vi "coler1.vi"(8 "error in":errorcluster, 11 "代刚":bool) -> (0 "error out":errorcluster)   [LabVIEW 2018]
uses:
  <vilib>/vision/NI_Vision_Development_Module.lvlib
panel:
  out "Array 3":dbl[](array[numeric])
  out "Color":u32(colorbox)
  out "Array":dbl[](array[numeric])
  out "Array 2":enum16{"黑", "紅", "黃", "綠", "藍"}[](array[ring])
  out "Image Out":T1(plugin-control)
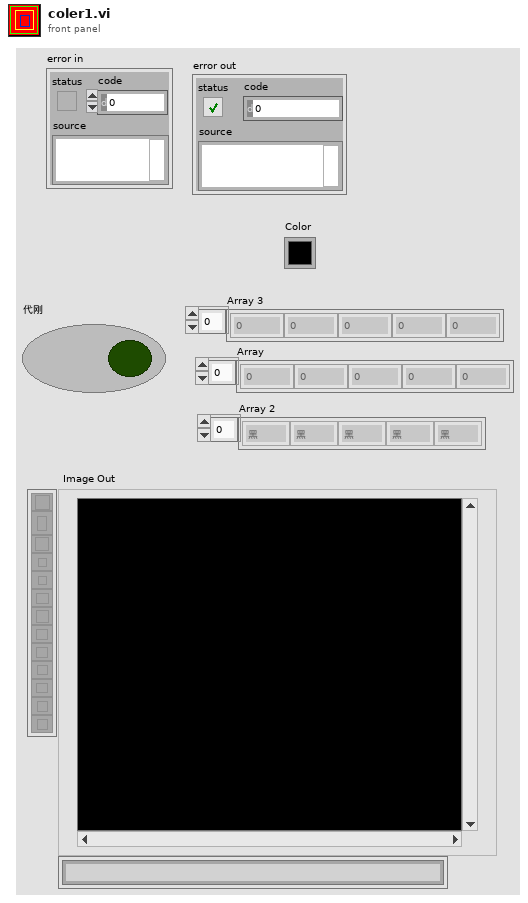
[diagram p1: front panel]
types:
  T1 = typedef "IMAQ Image.ctl" = refnum<image>
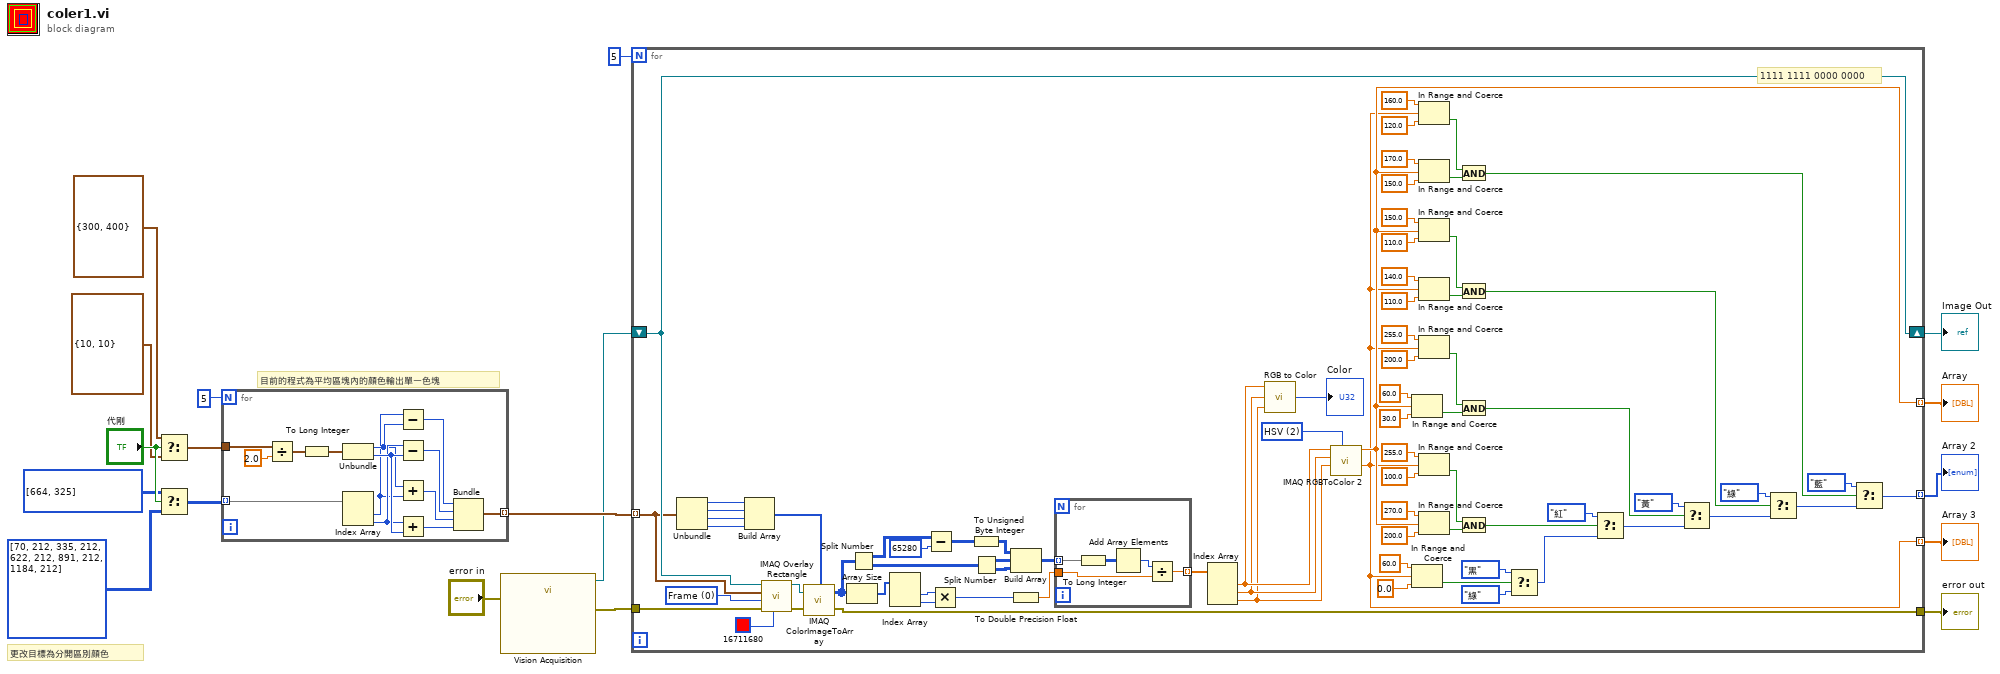
[diagram p0: block diagram]
diagram:
  # "更改目標為分開區別顏色"
  # "目前的程式為平均區塊內的顏色輸出單一色塊"
  n1 = Select(t=cluster{i32, i32} {300, 400}, s="代刚", f=cluster{i32, i32} {10, 10}) -> (s? t:f=w13:cluster{i32, i32})
  n2 = Select(t=i32[][] [[664, 325]], s="代刚", f=i32[][] [[70, 212], [335, 212], [622, 212], [891, 212], [1184, 212]]) -> (s? t:f=w14:i32[][])
  n3 = for {
    N: 5 -> [_]
    tunnel: w13 -> [w32]
    tunnel: w14 -> [w29] mode=indexing
    tunnel: [w19] -> w15 mode=indexing
    n4 = Divide(x=w32, y=2.0) -> (x/y=w30:cluster{dbl, dbl})
    n5 = To Long Integer(number=w30) -> (32bit integer=w28:cluster{i32, i32})
    n6 = Unbundle(w28) -> (w25:i32, w27:i32)
    n7 = Index Array(array=w29) -> (element #1=w24:i32, element #2=w26:i32)  [unwired: 2 in]
    n8 = Subtract(x=w24, y=w25) -> (x-y=w23:i32)
    n9 = Subtract(x=w26, y=w27) -> (x-y=w22:i32)
    n10 = Add(x=w25, y=w24) -> (x+y=w21:i32)
    n11 = Add(x=w26, y=w27) -> (x+y=w20:i32)
    n12 = Bundle(w23, w22, w21, w20) -> (w19:cluster{i32, i32, i32, i32})  [unwired: 1 in]
  }
  n13 = call "Vision Acquisition"("error in"="error in") -> ("Image Out"=w10:T1, "error out"=w12:errorcluster)  [unwired: 25 in]
  n14 = for {
    N: 5 -> [_]
    shift-right: [w87] -> w11
    shift-left: w10 -> [w87]
    tunnel: w12 -> [w89]
    tunnel: [w88] -> w18
    tunnel: w15 -> [w83] mode=indexing
    tunnel: [w64] -> w3 mode=indexing
    tunnel: [w59] -> w2 mode=indexing
    tunnel: [w33] -> w1 mode=indexing
    w94 = u16 2 items=["RGB", "HSL", "HSV", "HSI", "CIE L*a*b*", "CIE XYZ"] ("Color Mode")
    w109 = u32 0 items=["Frame", "Fill", "Highlight"] ("Drawing Mode (Frame)")
    # "1111 1111 0000 0000"
    n15 = Unbundle(w83) -> (w82:i32, w81:i32, w80:i32, w79:i32)
    n16 = Build Array(w82, w81, w80, w79) -> (w78:i32[])
    n17 = call "IMAQ Overlay Rectangle"("Color"=u32 16711680, "error in (no error)"=w89, "Drawing Mode (Frame)"=w109, "Rectangle"=w83, "Image"=w87) -> ("error out"=w85:errorcluster, "Image Out"=w86:T1)  [unwired: 5 in]
    n18 = call "IMAQ ColorImageToArray"("Optional Rectangle"=w78, "Image"=w86, "error in (no error)"=w85) -> ("Image Pixels (U32)"=w108:u32[][], "error out"=w88:errorcluster)  [unwired: 1 in, 1 out]
    n19 = Array Size(array=w108) -> (size(s)=w107:i32[])
    n20 = Split Number(x=w108) -> (hi(x)=w84:u16[][], lo(x)=w104:u16[][])
    n21 = Index Array(array=w107) -> (element #1=w98:i32, element #2=w99:i32)  [unwired: 2 in]
    n22 = Subtract(x=w84, y=u16 65280) -> (x-y=w105:u16[][])
    n23 = Multiply(x=w98, y=w99) -> (x*y=w97:i32)
    n24 = To Unsigned Byte Integer(number=w105) -> (unsigned 8bit integer=w103:u8[][])
    n25 = Split Number(x=w104) -> (hi(x)=w102:u8[][], lo(x)=w101:u8[][])
    n26 = Build Array(w103, w102, w101) -> (w100:u8[][][])
    n27 = To Double Precision Float(number=w97) -> (double precision float=w96:dbl)
    n28 = for {
      tunnel: w100 -> [w114] mode=indexing
      tunnel: w96 -> [w111]
      tunnel: [w110] -> w95 mode=indexing
      n29 = To Long Integer(number=w114) -> (32bit integer=w113:i32[][])
      n30 = Add Array Elements(numeric array=w113) -> (sum=w112:i32)
      n31 = Divide(x=w112, y=w111) -> (x/y=w110:dbl)
    }
    n32 = Index Array(array=w95) -> (element #1=w92:dbl, element #2=w91:dbl, element #3=w90:dbl)  [unwired: 3 in]
    n33 = call <vilib>:"RGB to Color.vi"("B"=w90, "G"=w91, "R"=w92) -> ("Color"=→"Color":u32)
    n34 = call "IMAQ RGBToColor 2"("Color Mode"=w94, "Blue value"=w90, "Green value"=w91, "Red value"=w92) -> ("Blue or Luma or Val or Inten or Z or b*value"=w33:dbl, "Red or Hue or X or L* value"=w59:dbl)  [unwired: 4 in, 2 out]
    n35 = In Range and Coerce(upper limit=60.0, x=w59, lower limit=30.0) -> (In Range?=w55:bool)  [unwired: 1 out]
    n36 = In Range and Coerce(upper limit=60.0, x=w33, lower limit=0.0 ("y")) -> (In Range?=w57:bool)  [unwired: 1 out]
    n37 = In Range and Coerce(upper limit=160.0, x=w33, lower limit=120.0) -> (In Range?=w37:bool)  [unwired: 1 out]
    n38 = In Range and Coerce(upper limit=170.0, x=w59, lower limit=150.0) -> (In Range?=w36:bool)  [unwired: 1 out]
    n39 = In Range and Coerce(upper limit=150.0, x=w59, lower limit=110.0) -> (In Range?=w42:bool)  [unwired: 1 out]
    n40 = In Range and Coerce(upper limit=140.0, x=w33, lower limit=110.0) -> (In Range?=w41:bool)  [unwired: 1 out]
    n41 = In Range and Coerce(upper limit=255.0, x=w33, lower limit=200.0) -> (In Range?=w51:bool)  [unwired: 1 out]
    n42 = In Range and Coerce(upper limit=255.0, x=w33, lower limit=100.0) -> (In Range?=w47:bool)  [unwired: 1 out]
    n43 = In Range and Coerce(upper limit=270.0, x=w59, lower limit=200.0) -> (In Range?=w48:bool)  [unwired: 1 out]
    n44 = And(x=w37, y=w36) -> (x .and. y?=w38:bool)
    n45 = And(x=w42, y=w41) -> (x .and. y?=w43:bool)
    n46 = And(x=w51, y=w55) -> (x .and. y?=w50:bool)
    n47 = And(x=w47, y=w48) -> (x .and. y?=w44:bool)
    n48 = Select(t=enum16{"黑", "紅", "黃", "綠", "藍"}."黑", s=w57, f=enum16{"黑", "紅", "黃", "綠", "藍"}."綠") -> (s? t:f=w58:enum16{"黑", "紅", "黃", "綠", "藍"})
    n49 = Select(t=enum16{"黑", "紅", "黃", "綠", "藍"}."紅", s=w44, f=w58) -> (s? t:f=w62:enum16{"黑", "紅", "黃", "綠", "藍"})
    n50 = Select(t=enum16{"黑", "紅", "黃", "綠", "藍"}."黃", s=w50, f=w62) -> (s? t:f=w69:enum16{"黑", "紅", "黃", "綠", "藍"})
    n51 = Select(t=enum16{"黑", "紅", "黃", "綠", "藍"}."綠", s=w43, f=w69) -> (s? t:f=w68:enum16{"黑", "紅", "黃", "綠", "藍"})
    n52 = Select(t=enum16{"黑", "紅", "黃", "綠", "藍"}."藍", s=w38, f=w68) -> (s? t:f=w64:enum16{"黑", "紅", "黃", "綠", "藍"})
  }
  "Image Out" <- w11
  "Array 2" <- w3
  "error out" <- w18
  "Array" <- w2
  "Array 3" <- w1
